vi "input.vi"(8 "error in":errorcluster, 10 "data table in":T1, 11 "Profibus Module runtime in":refnum<class "Profibus Module runtime.lvclass">) -> (0 "error out":errorcluster, 2 "data table out":T1, 3 "Profibus Module runtime out":refnum<class "Profibus Module runtime.lvclass">)   [LabVIEW 2013, in "Profibus Module runtime.lvclass"]
doc: "Provides an interface for reading data from a module at runtime. While this interface performs no operations, a child should provide an override which may read from any open sessions, references, or interfaces."
uses:
  Profibus Module runtime.lvclass
  dynamic profibus/dynamic profibus.lvlib
  <vilib>/NI/Tag Bus/table/data table.lvlib
  <vilib>/NI/Tag Bus/table/data polymorphs/write one/write Array of U8.vi
  <vilib>/NI/Tag Bus/table/data table.ctl
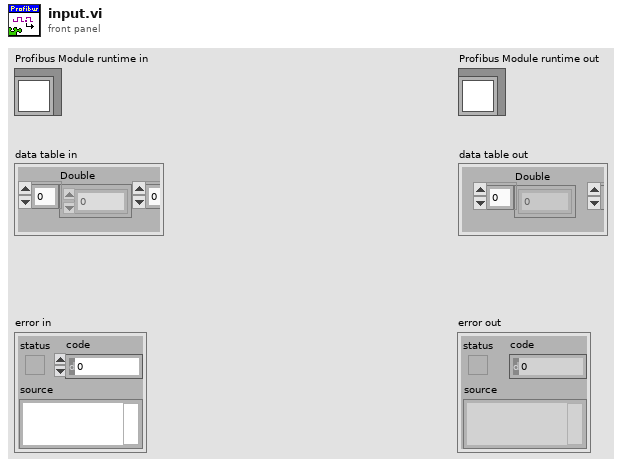
[diagram p1: front panel]
types:
  T1 = typedef "tag bus.lvlib/data table.lvlib/data table.ctl" = cluster{"Double":dbl[], "Single":sgl[], "I64":i64[], "I32":i32[], "I16":i16[], "I8":i8[], "U64":u64[], "U32":u32[], "U16":u16[], "U8":u8[], "Boolean":bool[], "String":string[], "Array of Double":cluster{"DBL Array":dbl[]}[], "Array of Single":cluster{"SGL Array":sgl[]}[], "Array of I64":cluster{"I64 Array":i64[]}[], "Array of I32":cluster{"I32 Array":i32[]}[], "Array of I16":cluster{"I16 Array":i16[]}[], "Array of I8":cluster{"I8 Array":i8[]}[], "Array of U64":cluster{"U64 Array":u64[]}[], "Array of U32":cluster{"U32 Array":u32[]}[], "Array of U16":cluster{"U16 Array":u16[]}[], "Array of U8":cluster{"U8 Array":u8[]}[], "Array of Boolean":cluster{"Boolean Array":bool[]}[], "Array of String":cluster{"String Array":string[]}[]}
  T2 = typedef "dynamic profibus.lvlib/fpga reference.ctl" = refnum<k20>
  T3 = typedef "Profibus Module runtime.lvclass/profibus slave configuration.ctl" = cluster{"slave index":i8, "data items":T4[], "data buffer":u8[], "big endian":bool, "data length":i32}
  T4 = typedef "Profibus Module runtime.lvclass/profibus mapping configuration.ctl" = cluster{"data type":T5, " byte":i32, " bit":i32, "tag index":i32}
  T5 = typedef "tag bus.lvlib/tag descriptor.lvclass/Data Type.ctl" = enum16{"Double", "Single", "I64", "I32", "I16", "I8", "U64", "U32", "U16", "U8", "Boolean", "String", "Array of Double", "Array of Single", "Array of I64", "Array of I32", "Array of I16", "Array of I8", "Array of U64", "Array of U32", "Array of U16", "Array of U8", "Array of Boolean", "Array of String"}
  T6 = enum16{"Start/Stop DP-Master", "Get Input Data", "Set Output Data", "Get Output Data", "Get Diagnostic Data", "Read/Write Data", "Read Diagnostic Data", "Get DPV1 Data", "Set DPV1 Data", "Read/Write DPV1 Data"}
  T7 = typedef "Profibus Module runtime.lvclass/profibus diagnostics reporting.ctl" = cluster{"slave":i8, "report":bool, "diagnostic tag":i32, "error specs":T8[]}
  T8 = typedef "Profibus Module configuration.lvclass/error throw specification.ctl" = cluster{"byte":i32, "bit":i32, "inverted?":bool, "error":i32}
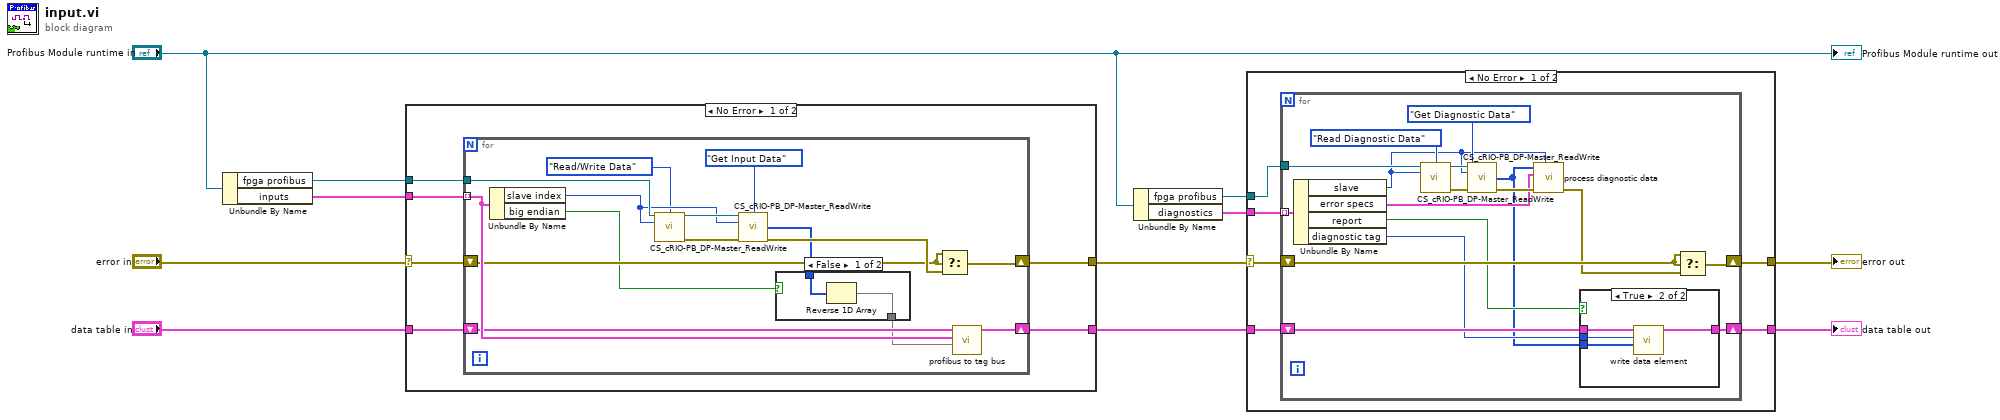
[diagram p0: block diagram]
diagram:
  n1 = Unbundle By Name("Profibus Module runtime in") -> ("fpga profibus"=w9:T2, "inputs"=w11:T3[])
  n2 = case shown="No Error" "error in" {
    selector: "error in" -> [w13 w37]
    tunnel: w11 -> [w17 _]
    tunnel: "data table in" -> [w16 w36]
    tunnel: [w15 w36] -> w4
    tunnel: w9 -> [w14 _]
    tunnel: [w12 w37] -> w7
    frame No Error {
      n3 = for {
        tunnel: w17 -> [w30] mode=indexing
        shift-right: [w31] -> w15
        shift-left: w16 -> [w29]
        shift-right: [w27] -> w12
        shift-left: w13 -> [w26]
        tunnel: w14 -> [w23]
        n4 = Unbundle By Name(w30) -> ("slave index"=w22:i8, "big endian"=w20:bool)
        n5 = call "CS_cRIO-PB_DP-Master_ReadWrite.vi"("FPGA VI Reference"=w23, "Mode"=T6."Read/Write Data", "Slave"=w22) -> ("FPGA VI Reference out"=w24:T2, "Error out"=w25:errorcluster)  [unwired: 9 in, 2 out]
        n6 = call "CS_cRIO-PB_DP-Master_ReadWrite.vi"("FPGA VI Reference"=w24, "Mode"=T6."Get Input Data", "Slave"=w22, "Error"=w25) -> ("Data out"=w18:u8[], "Error out"=w28:errorcluster)  [unwired: 8 in, 2 out]
        n7 = case shown="False" w20 {
          tunnel: [w33 w35] -> w19
          tunnel: w18 -> [w34 w35]
          frame False {
            n8 = Reverse 1D Array(array=w34) -> (reversed array=w33:u8[])
          }
          frame True {
          }
        }
        n9 = Select(t=w26, s=w26, f=w28) -> (s? t:f=w27:errorcluster)
        n10 = call "profibus to tag bus.vi"("Data in"=w19, "slave configuration"=w30, "data table in"=w29) -> ("data table out"=w31:T1)  [unwired: 8 in]
      }
    }
    frame Error {
    }
  }
  n11 = Unbundle By Name("Profibus Module runtime in") -> ("fpga profibus"=w2:T2, "diagnostics"=w1:T7[])
  n12 = case shown="No Error" w7 {
    selector: w7 -> [w41 w67]
    tunnel: [w40 w67] -> w6
    tunnel: [w42 w66] -> w5
    tunnel: w4 -> [w43 w66]
    tunnel: w2 -> [w39 _]
    tunnel: w1 -> [w38 _]
    frame No Error {
      n13 = for {
        shift-right: [w46] -> w42
        shift-left: w43 -> [w47]
        shift-right: [w60] -> w40
        shift-left: w41 -> [w59]
        tunnel: w39 -> [w54]
        tunnel: w38 -> [w53] mode=indexing
        n14 = Unbundle By Name(w53) -> ("slave"=w49:i8, "error specs"=w50:T8[], "report"=w48:bool, "diagnostic tag"=w45:i32)
        n15 = call "CS_cRIO-PB_DP-Master_ReadWrite.vi"("FPGA VI Reference"=w54, "Mode"=T6."Read Diagnostic Data", "Slave"=w49) -> ("FPGA VI Reference out"=w57:T2, "Error out"=w56:errorcluster)  [unwired: 9 in, 2 out]
        n16 = call "CS_cRIO-PB_DP-Master_ReadWrite.vi"("FPGA VI Reference"=w57, "Mode"=T6."Get Diagnostic Data", "Slave"=w49, "Error"=w56) -> ("Data out"=w44:u8[], "Error out"=w51:errorcluster)  [unwired: 8 in, 2 out]
        n17 = call "process diagnostic data.vi"("expected slave"=w49, "error in"=w51, "error specs"=w50, "diagnostic bytes"=w44) -> ("error out"=w52:errorcluster)  [unwired: 7 in]
        n18 = case shown="True" w48 {
          tunnel: w47 -> [w61 w65]
          tunnel: [w61 w64] -> w46
          tunnel: w45 -> [_ w63]
          tunnel: w44 -> [_ w62]
          frame False {
          }
          frame True {
            n19 = call-poly <vilib>:"write data element.vi"("value"=w62, "index"=w63, "data table in"=w65) -> ("data table out"=w64:T1)  [unwired: 8 in]
          }
        }
        n20 = Select(t=w59, s=w59, f=w52) -> (s? t:f=w60:errorcluster)
      }
    }
    frame Error {
    }
  }
  "error out" <- w6
  "data table out" <- w5
  "Profibus Module runtime out" <- "Profibus Module runtime in"
